vi "Eurotherm - VISA Serial - Write Command.vi"(0 "VISA resource name":refnum<visa-resource-name>, 2 "Read Reply":bool, 7 "write buffer":string, 11 "error in (no error)":errorcluster, 13 "Address":T1=1 min=1 max=99) -> (4 "dup VISA resource name":refnum<visa-resource-name>, 8 "bytes written":u32, 15 "error out":errorcluster)   [LabVIEW 2011]
uses:
  Eurotherm - Controls/Eurotherm - Address.ctl
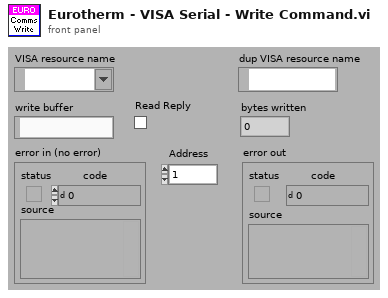
[diagram p1: front panel]
types:
  T1 = typedef "Eurotherm - Address.ctl" = u8
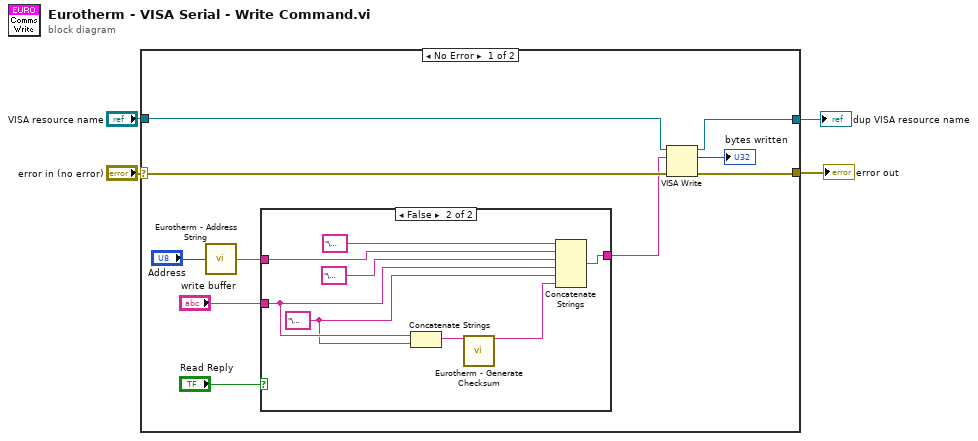
[diagram p0: block diagram]
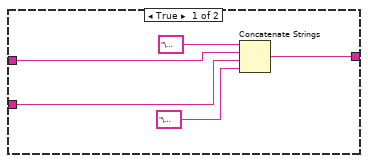
[diagram p2: hidden frame]
diagram:
  n1 = case shown="No Error" "error in (no error)" {
    selector: "error in (no error)" -> [w13 w29]
    tunnel: [w14 w29] -> w3
    tunnel: "VISA resource name" -> [w12 w28]
    tunnel: [w11 w28] -> w1
    frame No Error {
      n2 = call "Eurotherm - Address String.vi"("Address"="Address") -> ("String"=w5:string)  [unwired: 14 in]
      n3 = case shown="False" "Read Reply" {
        tunnel: [w18 w26] -> w9
        tunnel: "write buffer" -> [w16 w24]
        tunnel: w5 -> [w15 w20]
        frame True {
          n4 = Concatenate Strings("\u0004", w15, w16, "\u0005") -> (w18:string)
        }
        frame False {
          w23 = "\u0003"
          n5 = Concatenate Strings(w24, w23) -> (w22:string)
          n6 = call "Eurotherm - Generate Checksum.vi"("String"=w22) -> ("Checksum Character"=w21:string)  [unwired: 13 in, 1 out]
          n7 = Concatenate Strings("\u0004", w20, "\u0002", w24, w23, w21) -> (w26:string)
        }
      }
      n8 = VISA Write(VISA resource name=w12, write buffer=w9, error in (no error)=w13) -> (VISA resource name out=w11:refnum<visa-resource-name>, return count=→"bytes written":u32, error out=w14:errorcluster)
    }
    frame Error {
    }
  }
  "error out" <- w3
  "dup VISA resource name" <- w1
